vi "NFC-Main.vi"() -> ()   [LabVIEW 2018]
uses:
  <vilib>/myRIO/Instrument Drivers/Onboard IO/I2C/typedefs/I2C User Configuration.ctl
  <vilib>/myRIO/Instrument Drivers/Onboard IO/I2C/typedefs/I2C Transfer Rate.ctl
  <vilib>/myRIO/Instrument Drivers/Onboard IO/I2C/typedefs/I2C Reference.ctl
  <vilib>/myRIO/Common/Instrument Driver Framework/Utilities/typedefs/myRIO Generic Hardware Reference.ctl
  <vilib>/myRIO/Common/Instrument Driver Framework/Utilities/typedefs/Hardware Version Enum.ctl
  <vilib>/myRIO/Common/Instrument Driver Framework/Utilities/typedefs/myRIO v1.0 Reference.ctl
  <vilib>/myRIO/Common/Instrument Driver Framework/Utilities/typedefs/Generic FPGA Reference.ctl
  <vilib>/myRIO/Common/Instrument Driver Framework/myRIO v1.0/I2C/typedefs/I2C Channels Enum.ctl
  <vilib>/myRIO/Instrument Drivers/Onboard IO/I2C/typedefs/I2C Configuration.ctl
  <vilib>/userdefined/High Color/nirio_resource_hc.ctl
  <vilib>/myRIO/Instrument Drivers/Onboard IO/DIO/typedefs/DIO Reference.ctl
  <vilib>/myRIO/Common/Instrument Driver Framework/myRIO v1.0/DIO/typedefs/DIO Channels List.ctl
  <vilib>/myRIO/Common/Instrument Driver Framework/myRIO v1.0/DIO/typedefs/DIO Channels Enum.ctl
  <vilib>/myRIO/Common/Instrument Driver Framework/myRIO v1.0/I2C/vis/myRIO v1.1 Open I2C.vi
  <vilib>/myRIO/Common/Instrument Driver Framework/myRIO v1.0/DIO/vis/myRIO v1.1 Open DIO.vi
  <vilib>/myRIO/Common/Instrument Driver Framework/Utilities/vis/Validate Channels.vi
  <vilib>/myRIO/Common/Instrument Driver Framework/myRIO v1.0/I2C/vis/myRIO v1.0 Reserve I2C.vi
  <vilib>/myRIO/Common/Instrument Driver Framework/myRIO v1.0/DIO/vis/myRIO v1.0 Reserve DIO.vi
  <vilib>/myRIO/Common/Instrument Driver Framework/myRIO v1.0/I2C/vis/myRIO v1.0 Close I2C.vi
  <vilib>/myRIO/Common/Instrument Driver Framework/myRIO v1.0/DIO/vis/myRIO v1.0 Close DIO.vi
  <vilib>/myRIO/Common/Instrument Driver Framework/myRIO v1.0/I2C/vis/myRIO v1.0 Build MUX Configuration I2C.vi
  <vilib>/myRIO/Common/Instrument Driver Framework/myRIO v1.0/Resource Manager/vis/myRIO v1.0 Reserve Channel List.vi
  <vilib>/myRIO/Common/Instrument Driver Framework/myRIO v1.0/DIO/vis/myRIO v1.0 Build MUX Configuration DIO.vi
  <vilib>/myRIO/Common/Instrument Driver Framework/myRIO v1.0/I2C/vis/myRIO v1.0 Unreserve I2C.vi
  <vilib>/myRIO/Common/Instrument Driver Framework/myRIO v1.0/DIO/vis/myRIO v1.0 Unreserve DIO.vi
  <vilib>/myRIO/Common/Instrument Driver Framework/myRIO v1.0/Resource Manager/vis/myRIO v1.0 Create Configuration List.vi
  <vilib>/myRIO/Common/Instrument Driver Framework/myRIO v1.0/Resource Manager/vis/myRIO v1.0 Reserve Channel.vi
  <vilib>/myRIO/Common/Instrument Driver Framework/myRIO v1.0/Resource Manager/vis/myRIO v1.0 Unreserve Channel.vi
  <vilib>/myRIO/Common/Instrument Driver Framework/myRIO v1.0/Resource Manager/vis/myRIO v1.0 Unreserve Channel List.vi
  <vilib>/myRIO/Common/Instrument Driver Framework/myRIO v1.0/Resource Manager/vis/myRIO v1.0 Build Mutex Name.vi
  <vilib>/Utility/VariantDataType/GetNumericInfo.vi
  <vilib>/Utility/error.llb/Error Cluster From Error Code.vi
  <vilib>/myRIO/Common/Instrument Driver Framework/myRIO v1.0/myRIO v1.1 Open.vi
  <vilib>/myRIO/Common/Instrument Driver Framework/Utilities/vis/IO Manager.vi
  <vilib>/myRIO/Common/Instrument Driver Framework/Utilities/vis/Configuration Manager.vi
  <vilib>/myRIO/Common/Instrument Driver Framework/myRIO v1.0/Resource Manager/vis/myRIO v1.0 Configure IO.vi
  <vilib>/myRIO/Common/Instrument Driver Framework/myRIO v1.0/myRIO v1.0 Close.vi
  <vilib>/myRIO/Common/Instrument Driver Framework/myRIO v1.0/I2C/vis/myRIO v1.0 Configure I2C.vi
  <vilib>/myRIO/Common/Instrument Driver Framework/myRIO v1.0/I2C/vis/myRIO v1.0 Read I2C.vi
  <vilib>/myRIO/Common/Instrument Driver Framework/myRIO v1.0/I2C/vis/myRIO v1.0 Shutdown I2C.vi
  <vilib>/myRIO/Common/Instrument Driver Framework/myRIO v1.0/DIO/vis/myRIO v1.0 Shutdown DIO.vi
  <vilib>/myRIO/Instrument Drivers/Onboard IO/I2C/vis/myRIO I2C Open.xnode
  <vilib>/myRIO/Instrument Drivers/Onboard IO/DIO/vis/myRIO DIO Open.xnode
  <vilib>/myRIO/Instrument Drivers/Onboard IO/I2C/I2C.lvlib
  <vilib>/myRIO/Instrument Drivers/Onboard IO/DIO/DIO.lvlib
panel:
  out "ACK data":u8[](array[numeric]) format="%02x"
  out "Timeout occured?":bool
  out "error out":errorcluster
  in  "Stop Button":bool
  out "UID":string
  out "# of tags":u8
  out "State":string
  out "ACK Config":bool
  out "Bytes Read Config":u8[](array[numeric]) format="%02x"
  out "Bytes Read":u8[](array[numeric]) format="%02x"
  # "NFC Test"
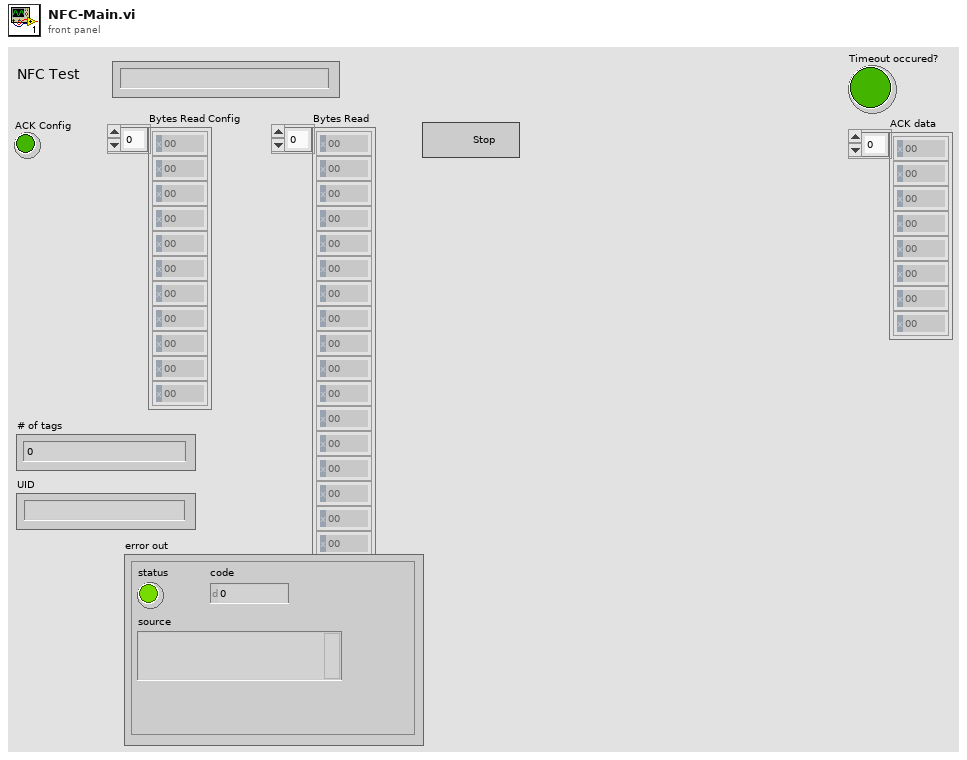
[diagram p1: front panel]
types:
  T1 = typedef "I2C.lvlib/I2C User Configuration.ctl" = cluster{"I2C Transfer Rate":T2}
  T2 = typedef "I2C.lvlib/I2C Transfer Rate.ctl" = enum16{"Standard mode (100 kbps)", "Fast mode (400 kbps)"}
  T3 = typedef "nirio_resource_hc.ctl" = tag
  T4 = typedef "Hardware Version Enum.ctl" = enum16{"Unknown", "myRIO-1900", "myRIO-1950", "roboRIO", "NI ELVIS RIO CM", "ELVIS III"}
  T5 = typedef "I2C.lvlib/I2C Reference.ctl" = cluster{"myRIO Reference":T6, "I2C Channels Enum":T9, "I2C Configuration":T10}
  T6 = typedef "myRIO Generic Hardware Reference.ctl" = cluster{"myRIO Model":T4, "myRIO Hardware Reference":T7}
  T7 = typedef "myRIO v1.0 Reference.ctl" = cluster{"Generic FPGA Reference":T8, "Allow multiple opens":bool}
  T8 = typedef "Generic FPGA Reference.ctl" = refnum<k20>
  T9 = typedef "I2C Channels Enum.ctl" = enum16{"Not Connected", "A/I2C", "B/I2C", "I2C/I2C"}
  T10 = typedef "I2C.lvlib/I2C Configuration.ctl" = cluster{"I2C Transfer Rate":T2}
  T11 = typedef "DIO.lvlib/DIO Reference.ctl" = cluster{"myRIO Reference":T6, "DIO Channels List":T12}
  T12 = typedef "DIO Channels List.ctl" = T13[]
  T13 = typedef "DIO Channels Enum.ctl" = enum16{"Not Connected", "C/DIO0", "C/DIO1", "C/DIO2", "C/DIO3", "C/DIO4", "C/DIO5", "C/DIO6", "C/DIO7", "A/DIO0", "A/DIO1", "A/DIO2", "A/DIO3", "A/DIO4", "A/DIO5", "A/DIO6", "A/DIO7", "A/DIO8", "A/DIO9", "A/DIO10", "A/DIO11", "A/DIO12", "A/DIO13", "A/DIO14", "A/DIO15", "A/DIO16", "A/DIO17", "A/DIO18", "A/DIO19", "B/DIO0", "B/DIO1", "B/DIO2", "B/DIO3", "B/DIO4", "B/DIO5", "B/DIO6", "B/DIO7", "B/DIO8", "B/DIO9", "B/DIO10", "B/DIO11", "B/DIO12", "B/DIO13", "B/DIO14", "B/DIO15", "B/DIO16", "B/DIO17", "B/DIO18", "B/DIO19", "LED0", "LED1", "LED2", "LED3", "Button0", "DIO/DIO0", "DIO/DIO1", "DIO/DIO2", "DIO/DIO3", "DIO/DIO4", "DIO/DIO5", "DIO/DIO6", "DIO/DIO7", "DIO/DIO8", "DIO/DIO9", "SPI/CS0", "SPI/CS1", "SPI/CS2", "SPI/CS3", "LED RADIO (Green)", "LED RADIO (Red)", "LED COMM (Green)", "LED COMM (Red)", "LED MODE (Green)", "LED MODE (Red)"}
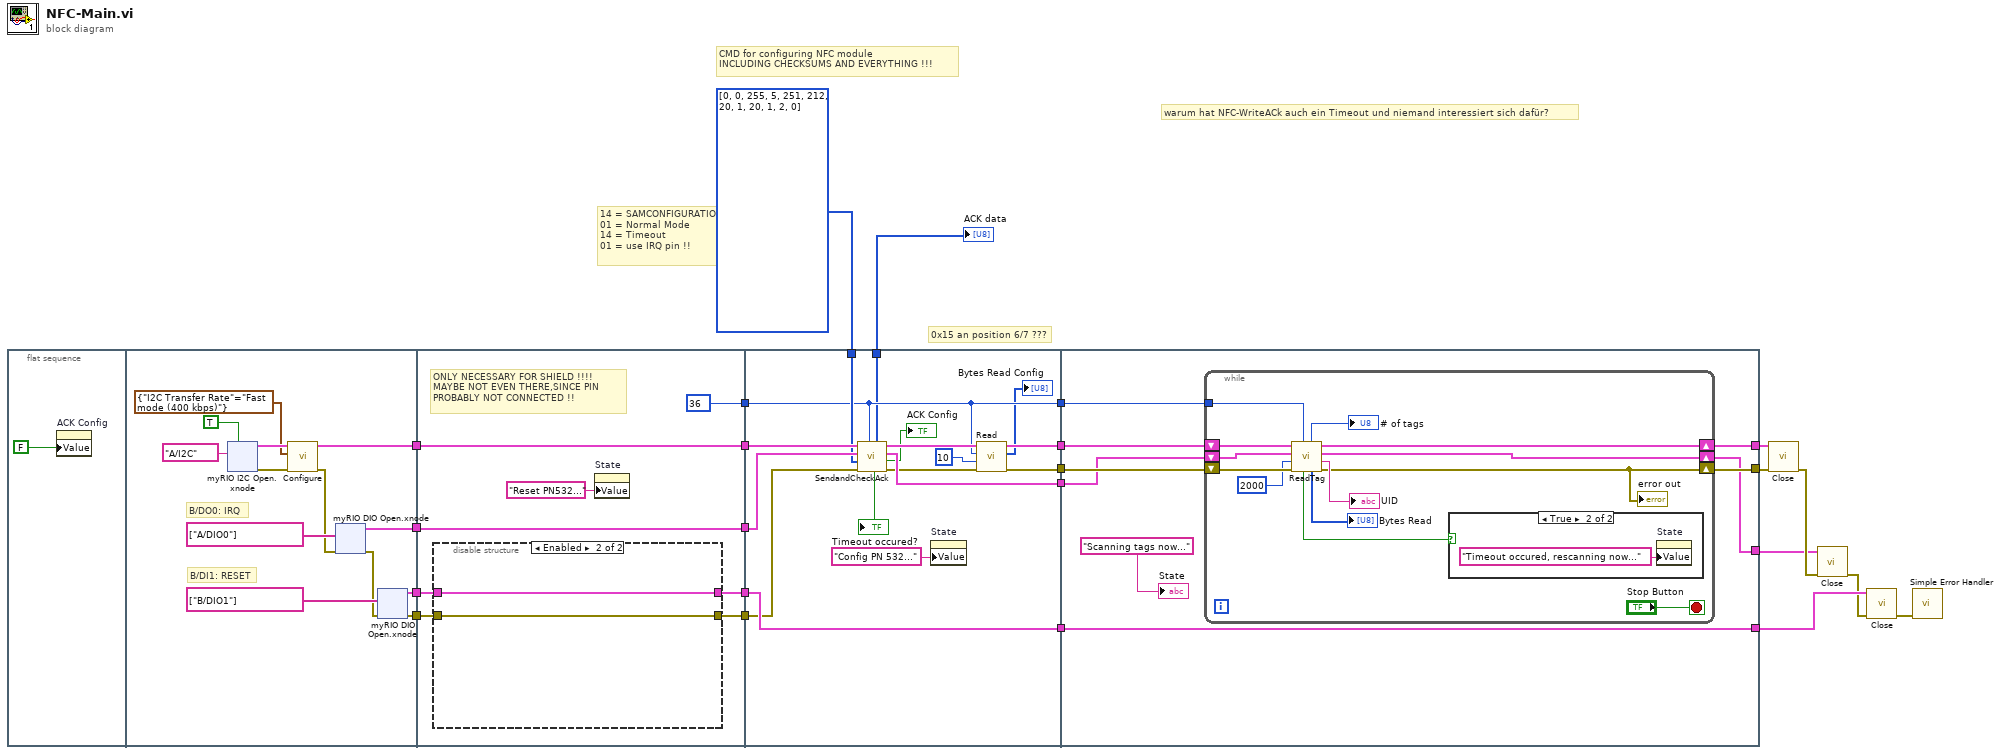
[diagram p0: block diagram]
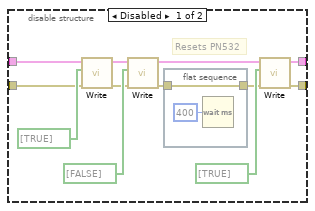
[diagram p2: hidden frame]
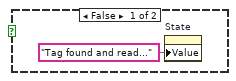
[diagram p3: hidden frame]
diagram:
  # "warum hat NFC-WriteACk auch ein Timeout und niemand interessiert sich dafür?"
  # "0x15 an position 6/7 ???"
  # "CMD for configuring NFC module\nINCLUDING CHECKSUMS AND EVERYTHING !!!"
  # "14 = SAMCONFIGURATION\n01 = Normal Mode\n14 = Timeout\n01 = use IRQ pin !!"
  n1 = flat-sequence {
    tunnel: [w33] -> w23
    tunnel: [w32] -> w22
    tunnel: [w31] -> w21
    tunnel: [w28] -> w20
    tunnel: w23 -> [w90]
    tunnel: w22 -> [w89]
    tunnel: w21 -> [w93]
    tunnel: w20 -> [w92]
    tunnel: [w87] -> w18
    tunnel: [u8 36 ("Slave Address (7-bit)")] -> w17
    tunnel: [w90] -> w16
    tunnel: [w89] -> w15
    tunnel: [w88] -> w13
    tunnel: w18 -> [w122]
    tunnel: w17 -> [w118]
    tunnel: w16 -> [w125]
    tunnel: w15 -> [w124]
    tunnel: [w123] -> w14
    tunnel: w13 -> [w126]
    tunnel: [w126] -> w12
    tunnel: [w118] -> w11
    tunnel: [w119] -> w10
    tunnel: u8[] [0, 0, 255, 5, 251, 212, 20, 1, 20, 1, 2, 0] -> [w121]
    tunnel: [w115] -> w5
    tunnel: [w110] -> w1
    tunnel: w14 -> [w132]
    tunnel: w12 -> [w135]
    tunnel: [w135] -> w19
    tunnel: w11 -> [w131]
    tunnel: w10 -> [w133]
    tunnel: w5 -> [w134]
    tunnel: [w130] -> w4
    tunnel: [w129] -> w3
    tunnel: [w128] -> w2
    frame #0 {
      n2 = property on="ACK Config" class="Bool (strict)"("Value"=FALSE ("ACK Config")) -> ()  [unwired: 2 in, 2 out]
    }
    frame #1 {
      # "B/DI1: RESET"
      # "B/DO0: IRQ"
      n3 = xnode "myRIO I2C Open.xnode"("Allow multiple opens?"=TRUE, "Channel Name"=tag "A/I2C") -> ("error out"=w36:errorcluster, "I2C Ref Out"=w37:T5)  [unwired: 1 in]
      n4 = call <vilib>:"Configure.vi"("error in (no error)"=w36, "I2C User Configuration"=T1 {"I2C Transfer Rate"=enum."Fast mode (400 kbps)"}, "I2C Ref In"=w37) -> ("error out"=w27:errorcluster, "I2C Ref Out"=w33:T5)  [unwired: 7 in]
      n5 = xnode "myRIO DIO Open.xnode"("error in (no error)"=w27, "Channel Names"=tag[] ["A/DIO0"]) -> ("error out"=w26:errorcluster, "DIO Ref Out"=w32:T11)  [unwired: 1 in]
      n6 = xnode "myRIO DIO Open.xnode"("error in (no error)"=w26, "Channel Names"=tag[] ["B/DIO1"]) -> ("error out"=w28:errorcluster, "DIO Ref Out"=w31:T11)  [unwired: 1 in]
    }
    frame #2 {
      # "ONLY NECESSARY FOR SHIELD !!!!\nMAYBE NOT EVEN THERE,SINCE PIN\nPROBABLY NOT CONNECTED !!"
      n7 = disable-structure shown="Enabled" {
        disable-tunnel: w93 -> [w105 w109]
        disable-tunnel: w92 -> [w102 w108]
        disable-tunnel: [w95 w109] -> w88
        disable-tunnel: [w94 w108] -> w87
        frame Disabled {
          # "Resets PN532"
          n8 = call <vilib>:"Write.vi"("error in (no error)"=w102, "Values"=bool[] [TRUE], "DIO Ref In"=w105) -> ("error out"=w101:errorcluster, "DIO Ref Out"=w100:T11)  [unwired: 6 in]
          n9 = call <vilib>:"Write.vi"("error in (no error)"=w101, "Values"=bool[] [FALSE], "DIO Ref In"=w100) -> ("error out"=w99:errorcluster, "DIO Ref Out"=w97:T11)  [unwired: 6 in]
          n10 = flat-sequence {
            tunnel: w99 -> [w107]
            tunnel: [w107] -> w96
            frame #0 {
              n11 = Wait (ms)(milliseconds to wait=u32 400) -> ()  [unwired: 1 out]
            }
          }
          n12 = call <vilib>:"Write.vi"("error in (no error)"=w96, "Values"=bool[] [TRUE], "DIO Ref In"=w97) -> ("error out"=w94:errorcluster, "DIO Ref Out"=w95:T11)  [unwired: 6 in]
        }
        frame Enabled {
        }
      }
      n13 = property on="State" class="Str"("Value"="Reset PN532..." ("State")) -> ()  [unwired: 2 in, 2 out]
    }
    frame #3 {
      n14 = call "SendandCheckAck.vi"("Slave Address (7-bit)"=w118, "error in (no error)"=w122, "bytes to send"=w121, "DI Ref In"=w124, "I2C Ref In"=w125) -> ("error out"=w117:errorcluster, "ACK?"=→"ACK Config":bool, "DI Ref Out"=w123:T11, "I2C Ref Out"=w120:T5, "Timeout occured?"=→"Timeout occured?":bool, "ACK data"=w110:u8[])  [unwired: 1 in]
      n15 = property on="State" class="Str"("Value"="Config PN 532..." ("State")) -> ()  [unwired: 2 in, 2 out]
      n16 = call <vilib>:"Read.vi"("error in (no error)"=w117, "Byte Count"=u32 10, "Slave Address (7-bit)"=w118, "I2C Ref In"=w120) -> ("error out"=w115:errorcluster, "Bytes Read"=→"Bytes Read Config":u8[], "I2C Ref Out"=w119:T5)  [unwired: 4 in]
    }
    frame #4 {
      n17 = while {
        tunnel: w131 -> [w145]
        shift-right: [w139] -> w129
        shift-left: w134 -> [w148]
        shift-right: [w140] -> w130
        shift-left: w133 -> [w147]
        shift-right: [w138] -> w128
        shift-left: w132 -> [w146]
        stop <- "Stop Button" stop-if-true
        n18 = call "ReadTag.vi"("Slave Address (7-bit)"=w145, "error in (no error)"=w148, "Timeout (ms)"=2000 ("Timeout (n-times 10 ms)"), "DI Ref Out"=w146, "I2C Ref Out in"=w147) -> ("error out"=w139:errorcluster, "UID"=→"UID":string, "DIO Ref Out out"=w138:T11, "I2C Ref Out out"=w140:T5, "Bytes Read"=→"Bytes Read":u8[], "# of tags"=→"# of tags":u8, "Timeout READ"=w137:bool)
        "error out" <- w139
        n19 = case shown="True" w137 {
          frame False {
            n20 = property on="State" class="Str"("Value"="Tag found and read..." ("State")) -> ()  [unwired: 2 in, 2 out]
          }
          frame True {
            n21 = property on="State" class="Str"("Value"="Timeout occured, rescanning now..." ("State")) -> ()  [unwired: 2 in, 2 out]
          }
        }
      }
      "State" <- "Scanning tags now..." ("State")
    }
  }
  n22 = call <vilib>:"Close.vi"("error in (no error)"=w3, "I2C Ref In"=w4) -> ("error out"=w9:errorcluster)  [unwired: 9 in]
  n23 = call <vilib>:"Close.vi"("error in (no error)"=w9, "DIO Ref In"=w2) -> ("error out"=w8:errorcluster)  [unwired: 9 in]
  n24 = call <vilib>:"Close.vi"("error in (no error)"=w8, "DIO Ref In"=w19) -> ("error out"=w7:errorcluster)  [unwired: 9 in]
  n25 = call <vilib>:"Simple Error Handler.vi"("error in (no error)"=w7) -> ()  [unwired: 4 in, 5 out]
  "ACK data" <- w1
